vi "Get Ctrl Refnum.vi"(8 "error in (no error)":errorcluster, 11 "Composed Field in":refnum<class "Composed Field.lvclass">) -> (0 "error out":errorcluster, 2 "Ctl Refnum":refnum<vi>, 3 "Composed Field out":refnum<class "Composed Field.lvclass">)   [LabVIEW 2020, in "Composed Fields.lvlib" / "Composed Field.lvclass"]
uses:
  Composed Field.lvclass
  C:/Users/User/Desktop/Raman Program/Database OOP/source/Database OOP/Column Libraries/Column/Composed Column.lvclass
  Reference Value Source/Reference Value Source.lvclass
  Column/Composed Column.lvclass/Composed Column.ctl
  Composed Columns/Value Source Interface Class/Value Source.lvclass
  Column/Composed Column.lvclass
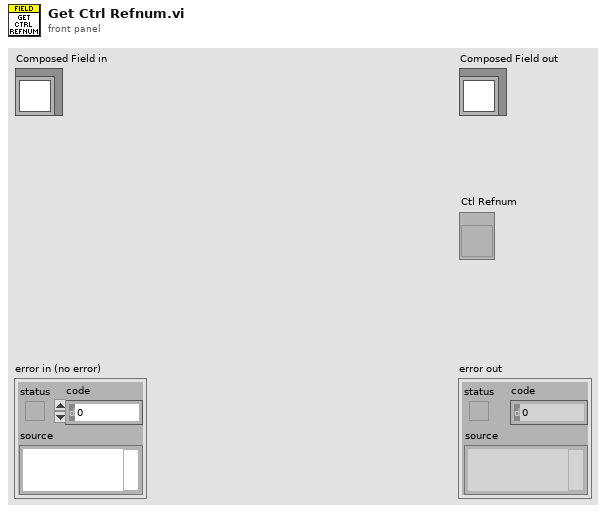
[diagram p1: front panel]
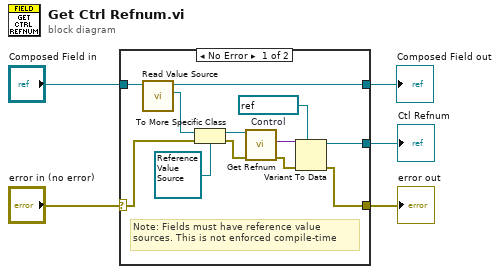
[diagram p0: block diagram]
diagram:
  n1 = case shown="No Error" "error in (no error)" {
    selector: "error in (no error)" -> [w14 w19]
    tunnel: [w6 w19] -> w4
    tunnel: "Composed Field in" -> [w17 w18]
    tunnel: [w13 w18] -> w2
    tunnel: [w7 _] -> w1
    frame No Error {
      w8 = refnum<vi> refnum  # Control
      # "Note: Fields must have reference value\nsources. This is not enforced compile-time"
      n2 = call "Read Value Source.vi"("Composed Column in"=w17) -> ("Value Source"=w16:refnum<class "Value Source.lvclass">, "Composed Column out"=w13:refnum<class "Composed Field.lvclass">)  [unwired: 8 in, 1 out]
      n3 = To More Specific Class(target class=refnum<class "Reference Value Source.lvclass"> refnum ("Composed Columns.lvlib:Reference Value Source.lvclass"), reference=w16, error in=w14) -> (specific class reference=w12:refnum<class "Reference Value Source.lvclass">, error out=w11:errorcluster)
      n4 = call-dynamic "Get Refnum.vi"("error in (no error)"=w11, "Reference Value Source in"=w12) -> ("error out"=w9:errorcluster, "Refnum"=w10:variant)  [unwired: 7 in, 1 out]
      n5 = Variant To Data(error in=w9, type=w8, Variant=w10) -> (data=w7:refnum<vi>, error out=w6:errorcluster)
    }
    frame Error {
    }
  }
  "error out" <- w4
  "Composed Field out" <- w2
  "Ctl Refnum" <- w1
